vi "Write Interface.lvclass.vi"(8 "error in (no error)":errorcluster, 10 "Interface.lvclass":refnum<class "Interface.lvclass">, 11 "Simulated_CCD_Camera in":refnum<class "Simulated_CCD_Camera.lvclass">) -> (0 "error out":errorcluster, 3 "Simulated_CCD_Camera out":refnum<class "Simulated_CCD_Camera.lvclass">)   [LabVIEW 2018, in "Simulated_CCD_Camera.lvclass"]
uses:
  Simulated_CCD_Camera.lvclass
  Interface/Interface.lvclass
  Simulated_CCD_Camera.lvclass/Simulated_CCD_Camera.ctl
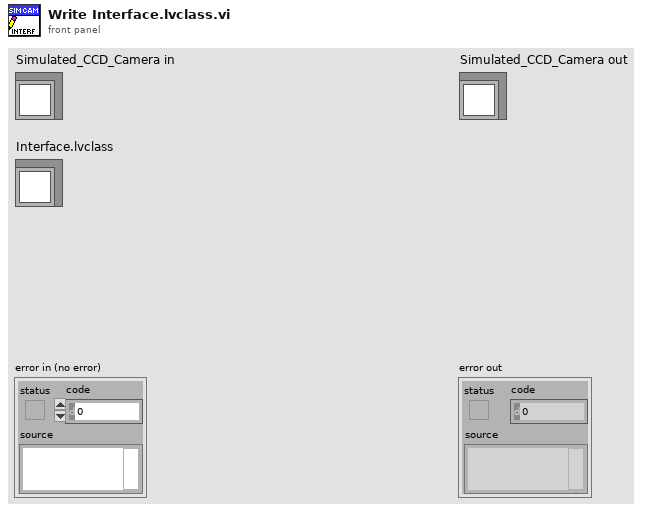
[diagram p1: front panel]
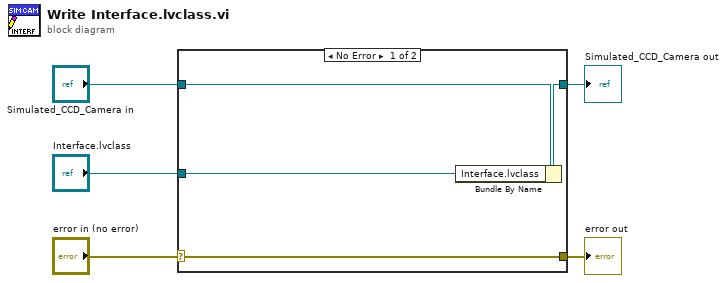
[diagram p0: block diagram]
diagram:
  n1 = case shown="No Error" "error in (no error)" {
    selector: "error in (no error)" -> [w9 w10]
    tunnel: [w9 w10] -> w4
    tunnel: [w7 w11] -> w2
    tunnel: "Simulated_CCD_Camera in" -> [w8 w11]
    tunnel: "Interface.lvclass" -> [w6 _]
    frame No Error {
      n2 = Bundle By Name(cluster=w8, "Interface.lvclass"=w6) -> (w7:refnum<class "Simulated_CCD_Camera.lvclass">)
    }
    frame Error {
    }
  }
  "error out" <- w4
  "Simulated_CCD_Camera out" <- w2
